vi "Build Message.vi"(6 "Value":dbl, 7 "Command":T2, 8 "error in":errorcluster, 11 "Luminos in":refnum<class "Luminos.lvclass">) -> (0 "error out":errorcluster, 2 "Message":T1={"Device Number"=0, "Command"=0, "Data"=0, "Response Count"=1} {"Command" items=["Echo"=55, "Home"=1, "Move Absolute"=20, "Move Relative"=21, "Move at Constant Speed"=22, "Renumber"=2, "Restore Settings"=36, "Stop"=23]}, 3 "Luminos out":refnum<class "Luminos.lvclass">)   [LabVIEW 2018, in "Luminos.lvlib" / "Luminos.lvclass"]
uses:
  Luminos.lvclass
  PPLs/Axis/Axis.lvlibp/Custom Controls/Command.ctl
  <instrlib>/ZaberTSeries/Public/Utility/Request.ctl
  Custom Controls/Command.ctl
  Luminos.lvclass/Luminos.ctl
  <instrlib>/ZaberTSeries/ZaberTSeries.lvlib
  PPLs/Axis/Axis.lvlibp/Axis.lvclass
  Luminos.lvlib
  C:/Projects/LabVIEW/PPLs/Axis/Axis.lvlibp/Axis.lvclass
  PPLs/Axis/Axis.lvlibp
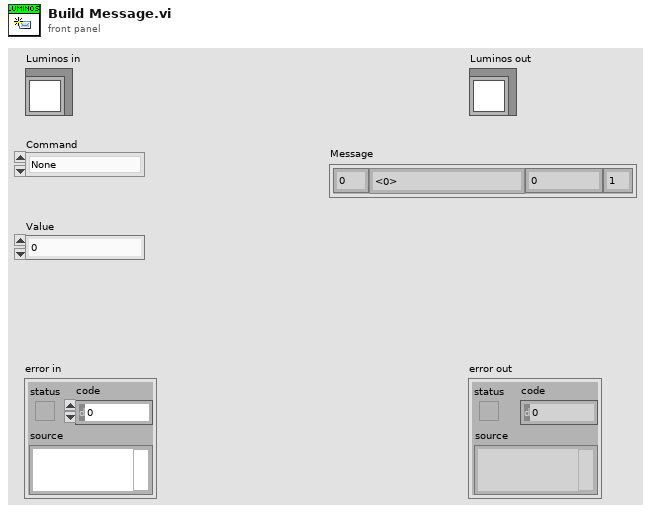
[diagram p1: front panel]
types:
  T1 = typedef "ZaberTSeries.lvlib/Request.ctl" = cluster{"Device Number":u8, "Command":u8, "Data":i32, "Response Count":i32}
  T2 = typedef "Axis.lvlibp/Command.ctl" = enum16{"None", "Home", "Renumber", "Move Absolute", "Move Relative", "Stop", "Set Run Speed", "Set Acceleration", "Set Run Current", "Set Home Offset", "Set Home Speed", "Query Current Position", "Load Defaults", "Query Status", "Lock Controls", "Unlock Controls"}
  T3 = typedef "Axis.lvlibp/Axis.ctl" = enum16{"None", "X", "Y", "Z", "Rx", "Ry", "Rz"}
  T4 = typedef "Luminos.lvlib/Command.ctl" = enum16{"None", "Home", "Renumber", "Move Absolute", "Move Relative", "Stop", "Set Run Speed", "Set Accel", "Set Run Current", "Set Home Offset", "Set Home Speed", "Current Position", "Load Defaults", "Status"}
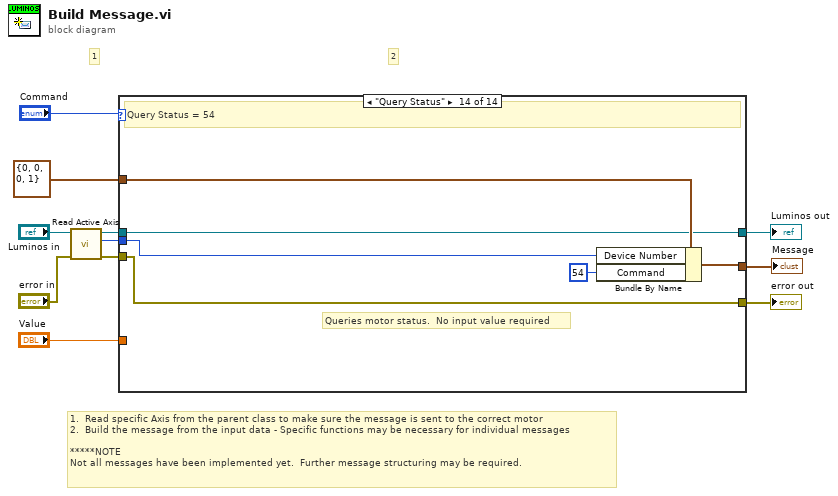
[diagram p0: block diagram]
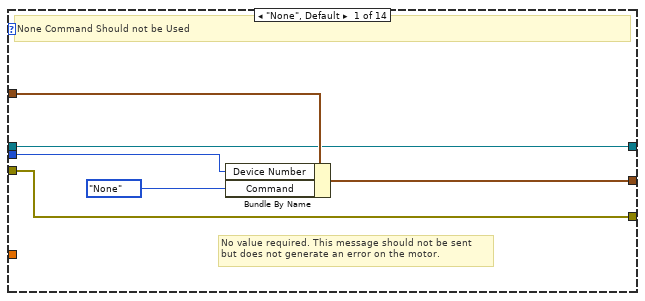
[diagram p2: hidden frame]
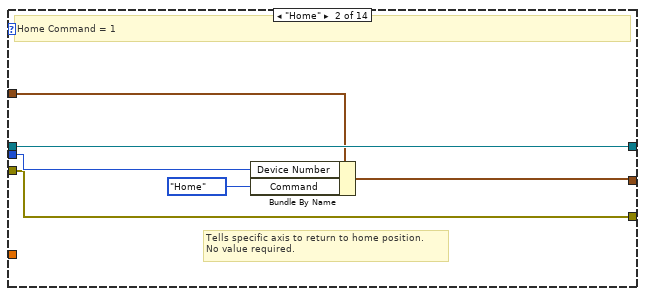
[diagram p3: hidden frame]
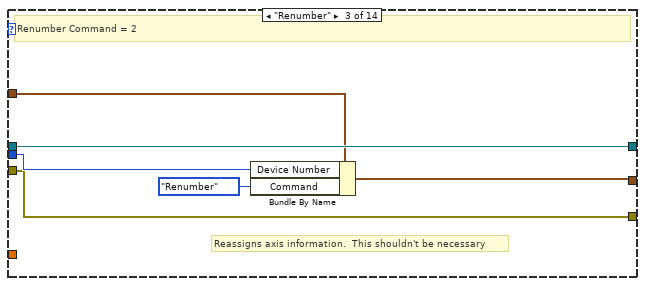
[diagram p4: hidden frame]
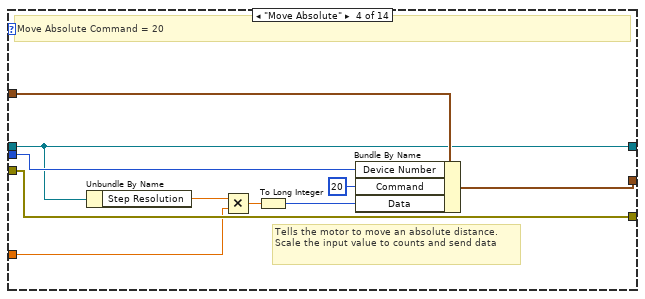
[diagram p5: hidden frame]
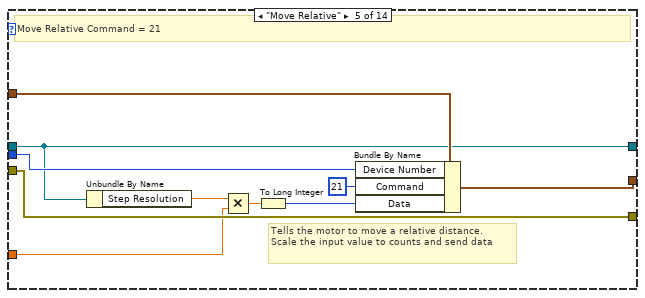
[diagram p6: hidden frame]
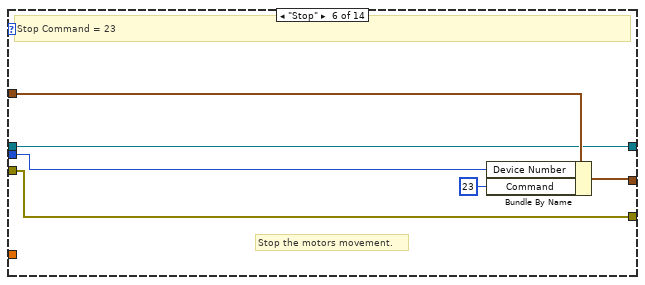
[diagram p7: hidden frame]
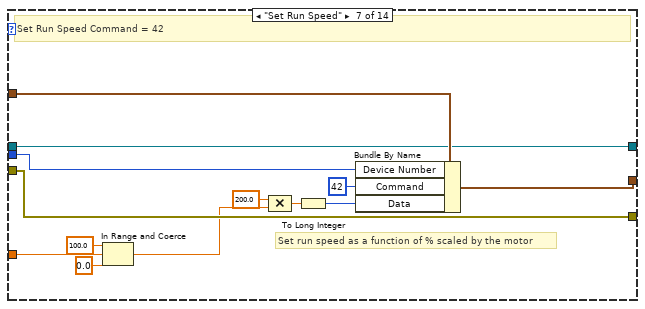
[diagram p8: hidden frame]
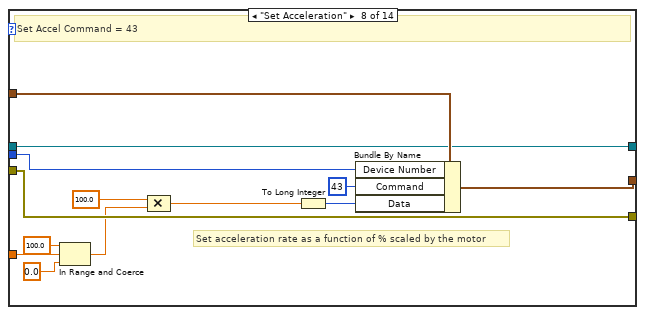
[diagram p9: hidden frame]
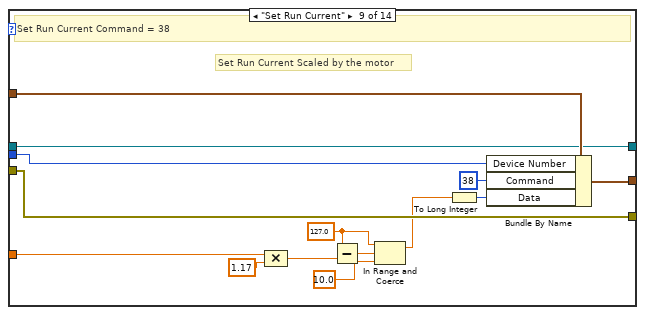
[diagram p10: hidden frame]
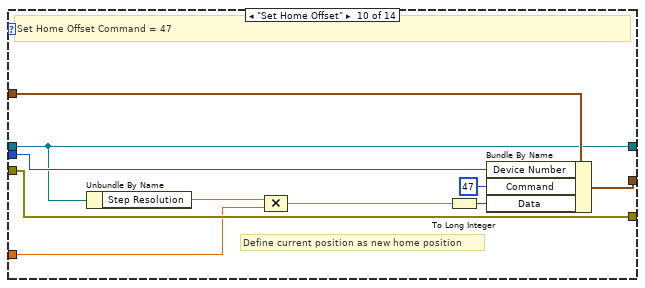
[diagram p11: hidden frame]
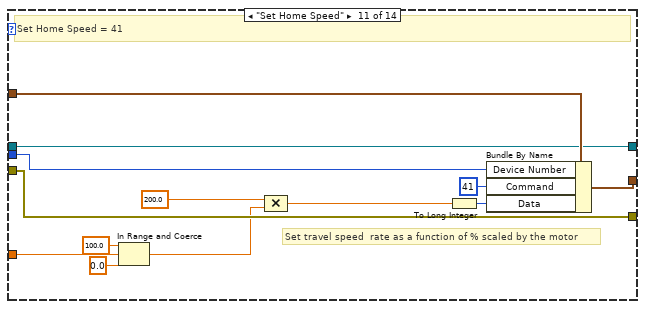
[diagram p12: hidden frame]
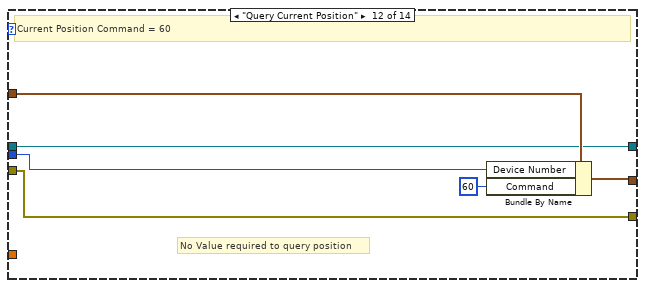
[diagram p13: hidden frame]
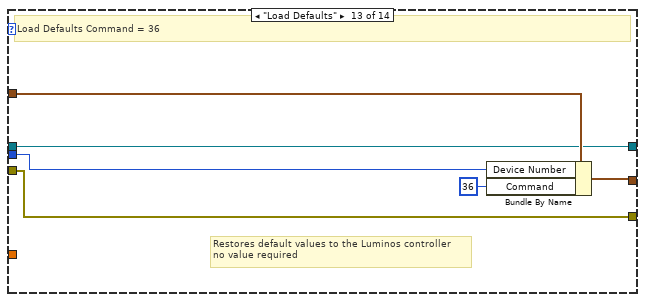
[diagram p14: hidden frame]
diagram:
  # "1.  Read specific Axis from the parent class to make sure the message is sent to the correct motor\n2.  Build the message from the input data - Specific functions may be necessary for individual messages\n\n*****NOTE\nNot all messages have been implemented yet.  Further message structuring may be required."
  # "2"
  # "1"
  n1 = call "Read Active Axis.vi"("error in"="error in", "Axis in"="Luminos in") -> ("error out"=w7:errorcluster, "Axis"=w8:T3, "Axis out"=w9:refnum<class "Luminos.lvclass">)  [unwired: 7 in]
  n2 = case shown="\"Query Status\"" "Command" {
    tunnel: w9 -> [w13 w23 w29 w35 w45 w51 w64 w77 w91 w101 w114 w120 w126 w132]
    tunnel: w8 -> [w15 w21 w27 w38 w48 w54 w67 w80 w94 w104 w117 w123 w129 w135]
    tunnel: w7 -> [w12 w18 w24 w36 w46 w52 w65 w78 w92 w102 w115 w121 w127 w133]
    tunnel: T1 {"Device Number"=0, "Command"=0, "Data"=0, "Response Count"=1} ("Message") -> [w17 w22 w28 w39 w49 w55 w68 w81 w95 w105 w118 w124 w130 w136]
    tunnel: [w16 w19 w25 w37 w47 w53 w66 w79 w93 w103 w116 w122 w128 w134] -> w5
    tunnel: [w13 w23 w29 w35 w45 w51 w64 w77 w91 w101 w114 w120 w126 w132] -> w4
    tunnel: [w12 w18 w24 w36 w46 w52 w65 w78 w92 w102 w115 w121 w127 w133] -> w2
    tunnel: "Value" -> [_ _ _ w33 w43 _ w61 w74 w88 w97 w111 _ _ _]
    frame "None", Default {
      # "No value required. This message should not be sent\nbut does not generate an error on the motor."
      # "None Command Should not be Used"
      n3 = Bundle By Name(cluster=w17, "Device Number"=w15, "Command"=Command."None") -> (w16:T1)
    }
    frame "Home" {
      # "Tells specific axis to return to home position.  \nNo value required."
      # "Home Command = 1"
      n4 = Bundle By Name(cluster=w22, "Device Number"=w21, "Command"=Command."Home") -> (w19:T1)
    }
    frame "Renumber" {
      # "Reassigns axis information.  This shouldn't be necessary"
      # "Renumber Command = 2"
      n5 = Bundle By Name(cluster=w28, "Device Number"=w27, "Command"=Command."Renumber") -> (w25:T1)
    }
    frame "Move Absolute" {
      # "Tells the motor to move an absolute distance. \nScale the input value to counts and send data"
      # "Move Absolute Command = 20"
      n6 = Unbundle By Name(w35) -> ("Step Resolution"=w34:dbl)
      n7 = Multiply(x=w34, y=w33) -> (x*y=w32:dbl)
      n8 = To Long Integer(number=w32) -> (32bit integer=w31:i32)
      n9 = Bundle By Name(cluster=w39, "Device Number"=w38, "Command"=u8 20, "Data"=w31) -> (w37:T1)
    }
    frame "Move Relative" {
      # "Tells the motor to move a relative distance. \nScale the input value to counts and send data"
      # "Move Relative Command = 21"
      n10 = Unbundle By Name(w45) -> ("Step Resolution"=w44:dbl)
      n11 = Multiply(x=w44, y=w43) -> (x*y=w42:dbl)
      n12 = To Long Integer(number=w42) -> (32bit integer=w41:i32)
      n13 = Bundle By Name(cluster=w49, "Device Number"=w48, "Command"=u8 21, "Data"=w41) -> (w47:T1)
    }
    frame "Stop" {
      # "Stop the motors movement."
      # "Stop Command = 23"
      n14 = Bundle By Name(cluster=w55, "Device Number"=w54, "Command"=u8 23) -> (w53:T1)
    }
    frame "Set Run Speed" {
      # "Set run speed as a function of % scaled by the motor"
      # "Set Run Speed Command = 42"
      n15 = In Range and Coerce(upper limit=100.0, x=w61, lower limit=0.0) -> (coerced(x)=w58:dbl)  [unwired: 1 out]
      n16 = Compound Arithmetic op=MULTIPLY(200.0 ("value"), w58) -> (w59:dbl)
      n17 = To Long Integer(number=w59) -> (32bit integer=w63:i32)
      n18 = Bundle By Name(cluster=w68, "Device Number"=w67, "Command"=u8 42, "Data"=w63) -> (w66:T1)
    }
    frame "Set Acceleration" {
      # "Set acceleration rate as a function of % scaled by the motor"
      # "Set Accel Command = 43"
      n19 = In Range and Coerce(upper limit=100.0, x=w74, lower limit=0.0) -> (coerced(x)=w71:dbl)  [unwired: 1 out]
      n20 = Compound Arithmetic op=MULTIPLY(100.0 ("value"), w71) -> (w72:dbl)
      n21 = To Long Integer(number=w72) -> (32bit integer=w76:i32)
      n22 = Bundle By Name(cluster=w81, "Device Number"=w80, "Command"=u8 43, "Data"=w76) -> (w79:T1)
    }
    frame "Set Run Current" {
      w83 = 127.0
      # "Set Run Current Scaled by the motor"
      # "Set Run Current Command = 38"
      n23 = Compound Arithmetic op=MULTIPLY(w88, 1.17 ("value")) -> (w85:dbl)
      n24 = Subtract(x=w83, y=w85) -> (x-y=w86:dbl)
      n25 = In Range and Coerce(upper limit=w83, x=w86, lower limit=10.0) -> (coerced(x)=w84:dbl)  [unwired: 1 out]
      n26 = To Long Integer(number=w84) -> (32bit integer=w90:i32)
      n27 = Bundle By Name(cluster=w95, "Device Number"=w94, "Command"=u8 38, "Data"=w90) -> (w93:T1)
    }
    frame "Set Home Offset" {
      # "Define current position as new home position"
      # "Set Home Offset Command = 47"
      n28 = Unbundle By Name(w101) -> ("Step Resolution"=w98:dbl)
      n29 = Compound Arithmetic op=MULTIPLY(w98, w97) -> (w96:dbl)
      n30 = To Long Integer(number=w96) -> (32bit integer=w100:i32)
      n31 = Bundle By Name(cluster=w105, "Device Number"=w104, "Command"=u8 47, "Data"=w100) -> (w103:T1)
    }
    frame "Set Home Speed" {
      # "Set travel speed  rate as a function of % scaled by the motor"
      # "Set Home Speed = 41"
      n32 = In Range and Coerce(upper limit=100.0, x=w111, lower limit=0.0) -> (coerced(x)=w108:dbl)  [unwired: 1 out]
      n33 = Compound Arithmetic op=MULTIPLY(200.0 ("value"), w108) -> (w110:dbl)
      n34 = To Long Integer(number=w110) -> (32bit integer=w113:i32)
      n35 = Bundle By Name(cluster=w118, "Device Number"=w117, "Command"=u8 41, "Data"=w113) -> (w116:T1)
    }
    frame "Query Current Position" {
      # "No Value required to query position"
      # "Current Position Command = 60"
      n36 = Bundle By Name(cluster=w124, "Device Number"=w123, "Command"=u8 60) -> (w122:T1)
    }
    frame "Load Defaults" {
      # "Restores default values to the Luminos controller\nno value required"
      # "Load Defaults Command = 36"
      n37 = Bundle By Name(cluster=w130, "Device Number"=w129, "Command"=u8 36) -> (w128:T1)
    }
    frame "Query Status" {
      # "Queries motor status.  No input value required"
      # "Query Status = 54"
      n38 = Bundle By Name(cluster=w136, "Device Number"=w135, "Command"=u8 54) -> (w134:T1)
    }
  }
  "error out" <- w2
  "Luminos out" <- w4
  "Message" <- w5
